vi "Power On.vi"(8 "error in (no error)":errorcluster, 11 "Dual Fan in":refnum<class "Dual Fan.lvclass">) -> (0 "error out":errorcluster, 3 "Dual Fan out":refnum<class "Dual Fan.lvclass">)   [LabVIEW 2012, in "Dual Fan.lvlib" / "Dual Fan.lvclass"]
uses:
  Dual Fan.lvclass
  Dual Fan.lvclass/Dual Fan.ctl
  Simulation/Simulation Data_Global.vi
  Simulation/Simulation.lvlib
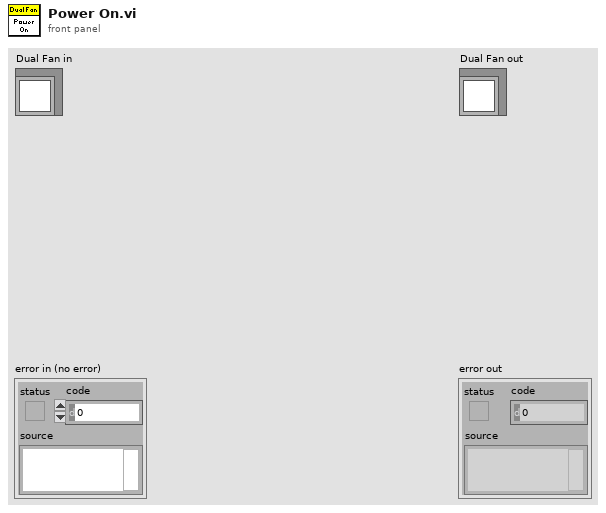
[diagram p1: front panel]
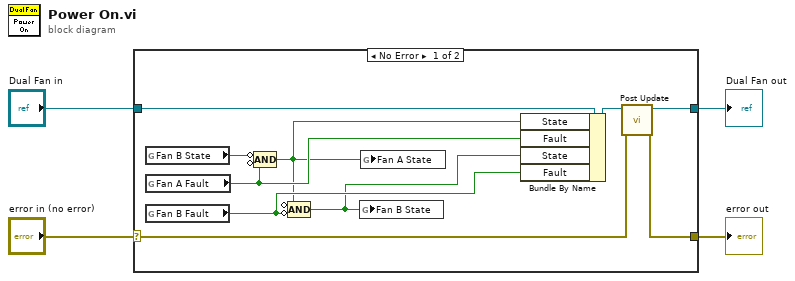
[diagram p0: block diagram]
diagram:
  n1 = case shown="No Error" "error in (no error)" {
    selector: "error in (no error)" -> [w5 w16]
    tunnel: [w11 w16] -> w3
    tunnel: [w12 w15] -> w1
    tunnel: "Dual Fan in" -> [w14 w15]
    frame No Error {
      n2 = global read "Simulation Data_Global.vi" "Fan B State"() -> (w8:bool)
      n3 = global read "Simulation Data_Global.vi" "Fan A Fault"() -> (w9:bool)
      n4 = global read "Simulation Data_Global.vi" "Fan B Fault"() -> (w10:bool)
      n5 = Compound Arithmetic op=AND(invert w8, invert w9) -> (w7:bool)
      n6 = Compound Arithmetic op=AND(invert w7, invert w10) -> (w6:bool)
      n7 = global write "Simulation Data_Global.vi" "Fan B State"(w6) -> ()
      n8 = global write "Simulation Data_Global.vi" "Fan A State"(w7) -> ()
      n9 = Bundle By Name(cluster=w14, "State"=w7, "Fault"=w9, "State"=w6, "Fault"=w10) -> (w13:refnum<class "Dual Fan.lvclass">)
      n10 = call "Post Update.vi"("error in (no error)"=w5, "Dual Fan in"=w13) -> ("error out"=w11:errorcluster, "Dual Fan out"=w12:refnum<class "Dual Fan.lvclass">)  [unwired: 8 in]
    }
    frame Error {
    }
  }
  "error out" <- w3
  "Dual Fan out" <- w1
